vi "Traffic signals using local variables.vi"() -> ()   [LabVIEW 2018]
panel:
  out "GREEN":bool
  out "YELLOW":bool
  out "RED":bool
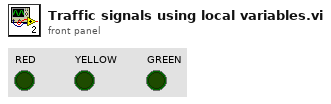
[diagram p1: front panel]
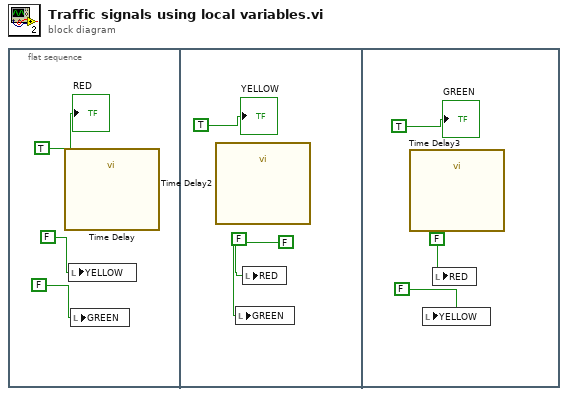
[diagram p0: block diagram]
diagram:
  n1 = flat-sequence {
    frame #0 {
      n2 = call "Time Delay"() -> ()  [unwired: 11 in, 1 out]
      n3 = local write "YELLOW"(FALSE) -> ()
      n4 = local write "GREEN"(FALSE) -> ()
      "RED" <- TRUE
    }
    frame #1 {
      n5 = call "Time Delay2"() -> ()  [unwired: 11 in, 1 out]
      n6 = local write "GREEN"(FALSE) -> ()
      n7 = local write "RED"(FALSE) -> ()
      "YELLOW" <- TRUE
    }
    frame #2 {
      n8 = call "Time Delay3"() -> ()  [unwired: 11 in, 1 out]
      n9 = local write "YELLOW"(FALSE) -> ()
      n10 = local write "RED"(FALSE) -> ()
      "GREEN" <- TRUE
    }
  }
